vi "overlay_positions.vi"(10 "Positions":cluster{"x":dbl, "y":dbl, "z":dbl}[](array[cluster]), 11 "Image":T1) -> (3 "Image 2":T1)   [LabVIEW 2010]
uses:
  <vilib>/vision/Image Controls.llb/IMAQ Image.ctl
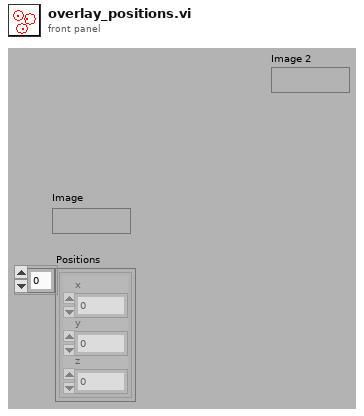
[diagram p1: front panel]
types:
  T1 = typedef "IMAQ Image.ctl" = refnum<image>
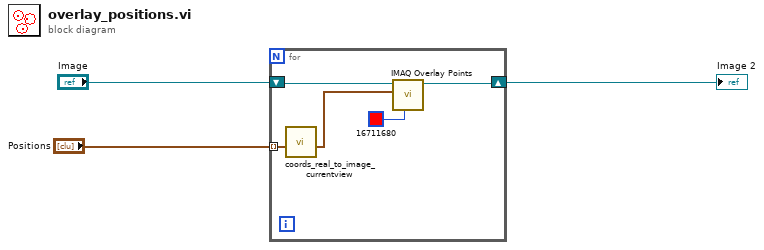
[diagram p0: block diagram]
diagram:
  n1 = for {
    shift-right: [w6] -> w1
    shift-left: "Image" -> [w8]
    tunnel: "Positions" -> [w5] mode=indexing
    n2 = call "coords_real_to_image_currentview.vi"("Position (real coords)"=w5) -> ("Position (pixels, relative to the top left of the image)"=w4:cluster{dbl, dbl})  [unwired: 7 in, 1 out]
    n3 = call "IMAQ Overlay Points"("Color"=u32 16711680, "Point"=w4, "Image"=w8) -> ("Image Out"=w6:T1)  [unwired: 7 in, 1 out]
  }
  "Image 2" <- w1
